vi "Single Item Save Dark Current.vi"(8 "Filename":string, 9 "Voltage":dbl, 10 "Barcode":string, 11 "Current":dbl) -> ()   [LabVIEW 2020]
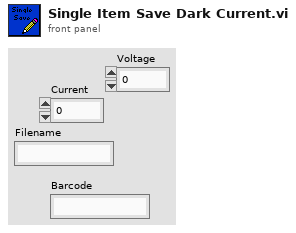
[diagram p1: front panel]
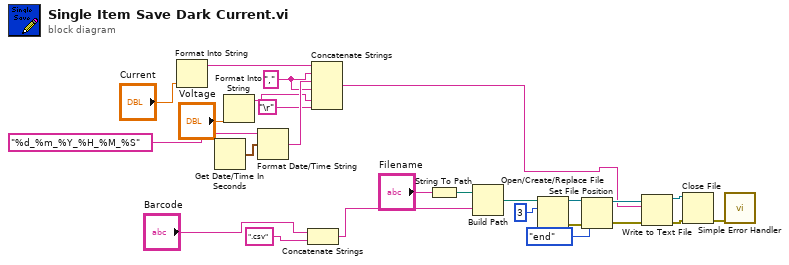
[diagram p0: block diagram]
diagram:
  w3 = ","
  n1 = Format Into String("Current") -> (resulting string=w24:string)  [unwired: 3 in, 1 out]
  n2 = Get Date/Time In Seconds() -> (seconds since 1Jan1904=w17:timestamp)
  n3 = Format Into String("Voltage") -> (resulting string=w1:string)  [unwired: 3 in, 1 out]
  n4 = Format Date/Time String(time format string (%c)="%d_%m_%Y_%H_%M_%S", seconds (now)=w17) -> (date/time string=w12:string)  [unwired: 1 in]
  n5 = Concatenate Strings("Barcode", ".csv" ("string")) -> (w13:string)
  n6 = Concatenate Strings(w24, w3, w12, w3, w1, "\r") -> (w6:string)
  n7 = String To Path(string="Filename") -> (path=w18:path)
  n8 = Build Path(base path=w18, name or relative path=w13) -> (appended path=w19:path)
  n9 = Open/Create/Replace File(file path (use dialog)=w19, operation (0:open)=3) -> (refnum out=w11:refnum<file>, error out=w10:errorcluster)  [unwired: 4 in, 1 out]
  n10 = Set File Position(refnum=w11, from (0:start)=enum16{"start", "end", "current"}."end", error in=w10) -> (refnum out=w8:refnum<file>, error out=w7:errorcluster)  [unwired: 1 in]
  n11 = Write to Text File(file (use dialog)=w8, text=w6, error in=w7) -> (refnum out=w20:refnum<file>, error out=w21:errorcluster)  [unwired: 1 in, 1 out]
  n12 = Close File(refnum=w20, error in=w21) -> (error out=w22:errorcluster)  [unwired: 1 out]
  n13 = call <vilib>:"Simple Error Handler.vi"("error in (no error)"=w22) -> ()  [unwired: 4 in, 5 out]
